vi "Config_Populate.vi"(8 "error in (no error)":errorcluster, 11 "Config Ref In":T1) -> (0 "error out":errorcluster, 3 "refnum out":T1)   [LabVIEW 2021]
uses:
  <vilib>/Utility/config.llb/Config Data RefNum.ctl
  Config_Cluster.ctl
  Mode_Enum.ctl
  <vilib>/Utility/config.llb/Write Key (Path).vi
  <vilib>/Utility/config.llb/Write Key (String).vi
  <vilib>/Utility/config.llb/Write Key (I32).vi
  <vilib>/Utility/config.llb/Write Key (Boolean).vi
  <vilib>/Utility/config.llb/NI_LVConfig.lvlib
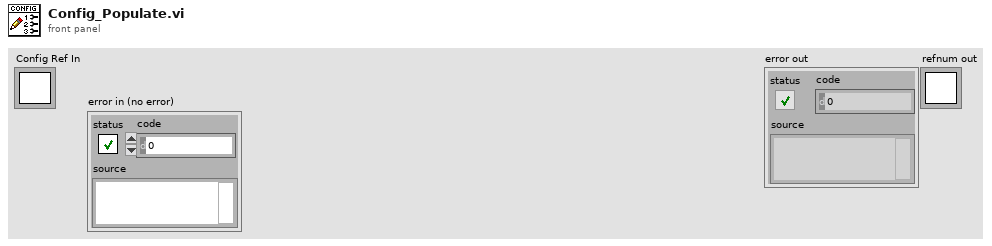
[diagram p1: front panel]
types:
  T1 = typedef "NI_LVConfig.lvlib/Config Data RefNum.ctl" = refnum<k1>
  T2 = typedef "Config_Cluster.ctl" = cluster{"General":cluster{"Config.ini":path, "Default Logging Path":path}, "Hardware":cluster{"LCR VISA COM":refnum<visa-resource-name>, "Measure Rate (1/s)":i32, "Reset on Load?":bool, "Measure Profile":path, "Global T VAR":refnum<k21>, "Global B VAR":refnum<k21>}, "HM8118 Current Profile":cluster{"Bias Profile":cluster{" Bias Source (OFF)":u8, " Bias Type (Voltage)":u8, "Bias Level (0)":dbl}, "Measurement Profile":cluster{"Operation Mode (0: Auto)":u16, "Circuit Type (2: Auto)":u16, "Manual Range (1:Range 1 and 25 Ohms)":u8, "Auto Range (T: Enable)":bool}, "Signal Profile":cluster{"Frequency (1kHz)":dbl, "Measuring Voltage (1V)":dbl}, "Integration Profile":cluster{"Averaging (0: Off)":u16, "Averaging Number (2)":i32, "Time (100ms)":i32, "Rate (0: Fast)":u16}, "Trigger Profile":cluster{"Trigger Mode (0: Continuous)":u16}}, "HM8118 New Profile":cluster{"Bias Profile":cluster{" Bias Source (OFF)":u8, " Bias Type (Voltage)":u8, "Bias Level (0)":dbl}, "Measurement Profile":cluster{"Operation Mode (0: Auto)":u16, "Circuit Type (2: Auto)":u16, "Manual Range (1:Range 1 and 25 Ohms)":u8, "Auto Range (T: Enable)":bool}, "Signal Profile":cluster{"Frequency (1kHz)":dbl, "Measuring Voltage (1V)":dbl}, "Integration Profile":cluster{"Averaging (0: Off)":u16, "Averaging Number (2)":i32, "Time (100ms)":i32, "Rate (0: Fast)":u16}, "Trigger Profile":cluster{"Trigger Mode (0: Continuous)":u16}}, "Operation":cluster{"Operation Mode":T3, "Status":string, "NewLog?":bool}}
  T3 = typedef "Mode_Enum.ctl" = enum16{"Logging", "Idle-Off", "Idle"}
  T4 = cluster{"Config.ini":path, "Default Logging Path":path}
  T5 = cluster{"LCR VISA COM":refnum<visa-resource-name>, "Measure Rate (1/s)":i32, "Reset on Load?":bool, "Measure Profile":path, "Global T VAR":refnum<k21>, "Global B VAR":refnum<k21>}
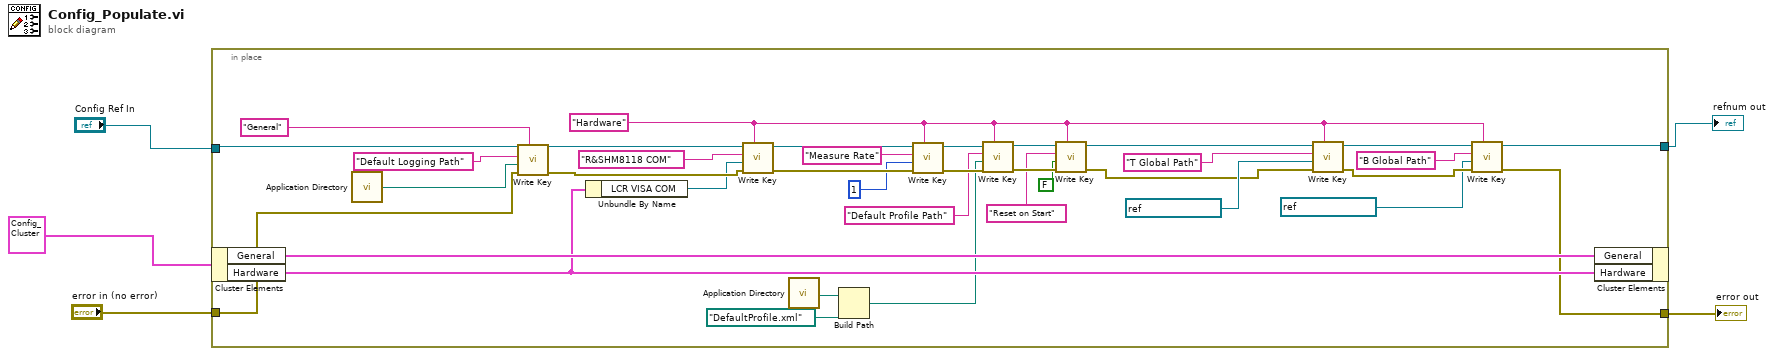
[diagram p0: block diagram]
diagram:
  n1 = in-place {
    in-place-border: "Config Ref In" -> [w41]
    in-place-border: "error in (no error)" -> [w40]
    in-place-border: [w6] -> w2
    in-place-border: [w7] -> w1
    w14 = "Hardware" ("section")
    n2 = in-place-cluster #1(T2 {"General"={"Config.ini"=path "", "Default Logging Path"=path ""}, "Hardware"={"LCR VISA COM"="", "Measure Rate (1/s)"=0, "Reset on Load?"=FALSE, "Measure Profile"=path "", "Global T VAR"="", "Global B VAR"=""}, "HM8118 Current Profile"={"Bias Profile"={" Bias Source (OFF)"=0, " Bias Type (Voltage)"=0, "Bias Level (0)"=0.0}, "Measurement Profile"={"Operation Mode (0: Auto)"=0, "Circuit Type (2: Auto)"=0, "Manual Range (1:Range 1 and 25 Ohms)"=0, "Auto Range (T: Enable)"=FALSE}, "Signal Profile"={"Frequency (1kHz)"=0.0, "Measuring Voltage (1V)"=0.0}, "Integration Profile"={"Averaging (0: Off)"=0, "Averaging Number (2)"=0, "Time (100ms)"=0, "Rate (0: Fast)"=0}, "Trigger Profile"={"Trigger Mode (0: Continuous)"=0}}, "HM8118 New Profile"={"Bias Profile"={" Bias Source (OFF)"=0, " Bias Type (Voltage)"=0, "Bias Level (0)"=0.0}, "Measurement Profile"={"Operation Mode (0: Auto)"=0, "Circuit Type (2: Auto)"=0, "Manual Range (1:Range 1 and 25 Ohms)"=0, "Auto Range (T: Enable)"=FALSE}, "Signal Profile"={"Frequency (1kHz)"=0.0, "Measuring Voltage (1V)"=0.0}, "Integration Profile"={"Averaging (0: Off)"=0, "Averaging Number (2)"=0, "Time (100ms)"=0, "Rate (0: Fast)"=0}, "Trigger Profile"={"Trigger Mode (0: Continuous)"=0}}, "Operation"={"Operation Mode"=enum."Logging", "Status"="", "NewLog?"=FALSE}} ("Configuration Cluster")) -> ("General"=w37:T4, "Hardware"=w36:T5)
    n3 = call <vilib>:"Application Directory.vi"() -> ("Application Directory"=w28:path)
    n4 = call-poly <vilib>:"Write Key.vi"("section"="General", "error in (no error)"=w40, "value"=w28, "key"="Default Logging Path", "refnum"=w41) -> ("error out"=w35:errorcluster, "refnum out"=w38:T1)  [unwired: 4 in, 1 out]
    n5 = Unbundle By Name(w36) -> ("LCR VISA COM"=w33:refnum<visa-resource-name>)
    n6 = call-poly <vilib>:"Write Key.vi"("section"=w14, "error in (no error)"=w35, "value"=w33, "key"="R&SHM8118 COM", "refnum"=w38) -> ("error out"=w30:errorcluster, "refnum out"=w31:T1)  [unwired: 4 in, 1 out]
    n7 = call <vilib>:"Application Directory.vi"() -> ("Application Directory"=w23:path)
    n8 = Build Path(base path=w23, name or relative path=path "DefaultProfile.xml") -> (appended path=w21:path)
    n9 = call-poly <vilib>:"Write Key.vi"("section"=w14, "error in (no error)"=w30, "value"=1 ("Measure Rate (1/s)"), "key"="Measure Rate", "refnum"=w31) -> ("error out"=w26:errorcluster, "refnum out"=w25:T1)  [unwired: 4 in, 1 out]
    n10 = call-poly <vilib>:"Write Key.vi"("section"=w14, "error in (no error)"=w26, "value"=w21, "key"="Default Profile Path", "refnum"=w25) -> ("error out"=w19:errorcluster, "refnum out"=w20:T1)  [unwired: 4 in, 1 out]
    n11 = call-poly <vilib>:"Write Key.vi"("section"=w14, "error in (no error)"=w19, "value"=FALSE, "key"="Reset on Start", "refnum"=w20) -> ("error out"=w11:errorcluster, "refnum out"=w16:T1)  [unwired: 4 in, 1 out]
    n12 = call-poly <vilib>:"Write Key.vi"("section"=w14, "error in (no error)"=w11, "value"=refnum<k21> "ni.var.psp://localhost/SV_Temperature/T_VTI_val" ("shared variable refnum in"), "key"="T Global Path", "refnum"=w16) -> ("error out"=w9:errorcluster, "refnum out"=w15:T1)  [unwired: 4 in, 1 out]
    n13 = call-poly <vilib>:"Write Key.vi"("section"=w14, "error in (no error)"=w9, "value"=refnum<k21> "ni.var.psp://localhost/SV_Magnet/B_an_val" ("shared variable refnum in"), "key"="B Global Path", "refnum"=w15) -> ("error out"=w6:errorcluster, "refnum out"=w7:T1)  [unwired: 4 in, 1 out]
    n14 = in-place-cluster #1("General"=w37, "Hardware"=w36) -> ()  [unwired: 1 out]
  }
  "error out" <- w2
  "refnum out" <- w1
